vi "DataFinder Find Run Results.vi"(10 "RUNSELECT (Most Recent, First, ALL)":string, 11 "Run Results (empty)":T1[](array[typedef])) -> (3 "Filtered Run Results":T1[](array[typedef]))   [LabVIEW 2011]
uses:
  www/cgi-bin/_cgi-lib/TDM_INDEX Record.ctl
  www/cgi-bin/_cgi-lib/TDM_INDEX Record text SN sort.ctl
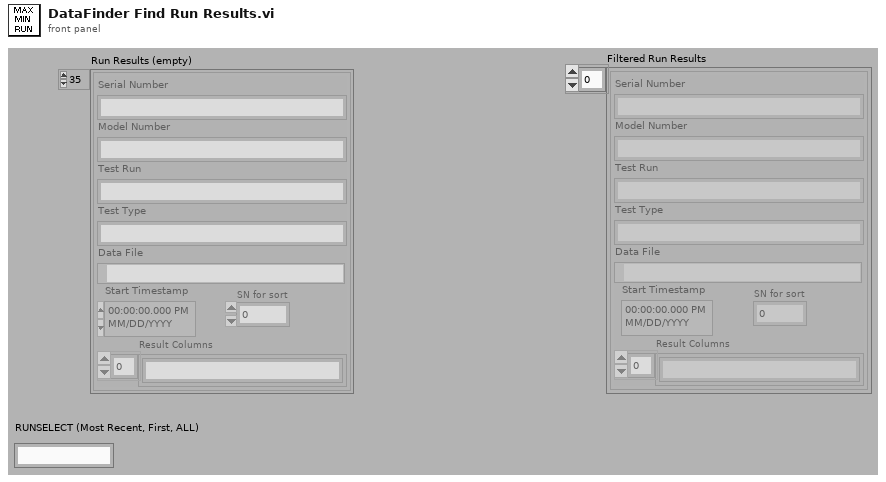
[diagram p1: front panel]
types:
  T1 = typedef "TDM_INDEX Record.ctl" = cluster{"Model Number":string, "SN for sort":i32, "Test Type":string, "Test Run":string, "Serial Number":string, "Start Timestamp":timestamp, "Data File":path, "Result Columns":string[]}
  T2 = typedef "TDM_INDEX Record text SN sort.ctl" = cluster{"Model Number":string, "Serial Number":string, "Test Type":string, "Test Run":string, "SN for sort":i32, "Start Timestamp":timestamp, "Data File":path, "Result Columns":string[]}
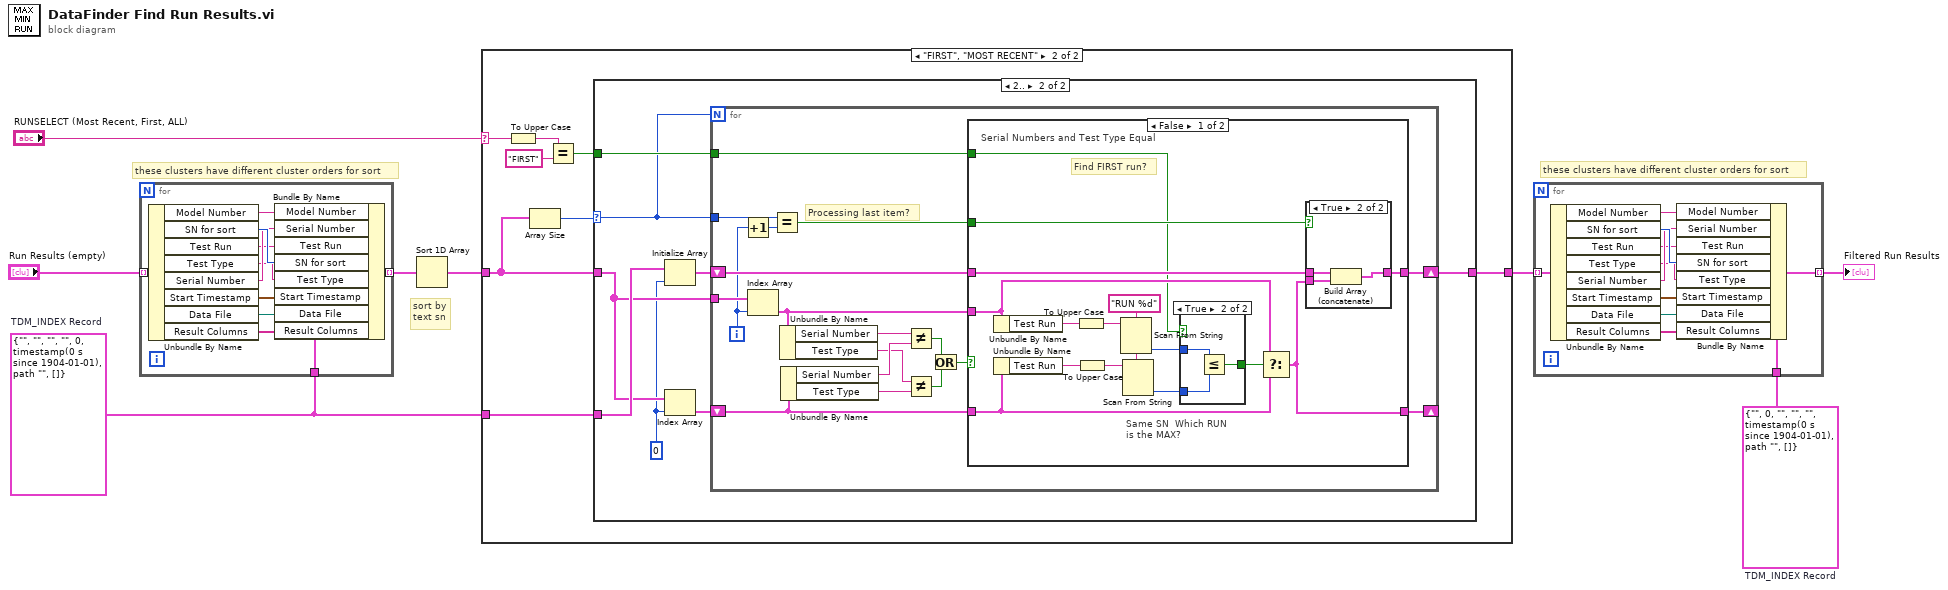
[diagram p0: block diagram]
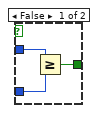
[diagram p4: hidden frame]
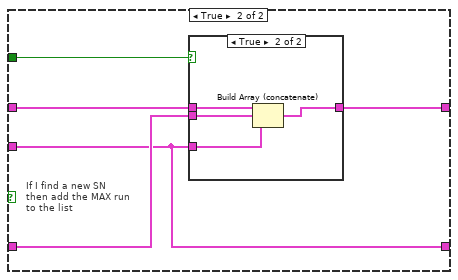
[diagram p6: hidden frame]
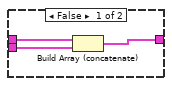
[diagram p7: hidden frame]
diagram:
  w3 = T1 {"Model Number"="", "SN for sort"=0, "Test Type"="", "Test Run"="", "Serial Number"="", "Start Timestamp"=timestamp(0 s since 1904-01-01), "Data File"=path "", "Result Columns"=[]}  # TDM_INDEX Record
  w6 = T2 {"Model Number"="", "Serial Number"="", "Test Type"="", "Test Run"="", "SN for sort"=0, "Start Timestamp"=timestamp(0 s since 1904-01-01), "Data File"=path "", "Result Columns"=[]}  # TDM_INDEX Record
  # "sort by\ntext sn"
  # "these clusters have different cluster orders for sort"
  # "these clusters have different cluster orders for sort"
  n1 = for {
    tunnel: "Run Results (empty)" -> [w19] mode=indexing
    tunnel: w6 -> [w18]
    tunnel: [w9] -> w5 mode=indexing
    n2 = Unbundle By Name(w19) -> ("Model Number"=w17:string, "SN for sort"=w16:i32, "Test Run"=w14:string, "Test Type"=w13:string, "Serial Number"=w15:string, "Start Timestamp"=w12:timestamp, "Data File"=w11:path, "Result Columns"=w10:string[])
    n3 = Bundle By Name(cluster=w18, "Model Number"=w17, "Serial Number"=w15, "Test Run"=w14, "SN for sort"=w16, "Test Type"=w13, "Start Timestamp"=w12, "Data File"=w11, "Result Columns"=w10) -> (w9:T2)
  }
  n4 = Sort 1D Array(array=w5) -> (sorted array=w4:T2[])
  n5 = case shown="\"FIRST\", \"MOST RECENT\"" "RUNSELECT (Most Recent, First, ALL)" {
    selector: "RUNSELECT (Most Recent, First, ALL)" -> [_ w24]
    tunnel: [w20 w28] -> w7
    tunnel: w4 -> [w20 w27]
    tunnel: w6 -> [_ w25]
    frame "ALL", Default {
    }
    frame "FIRST", "MOST RECENT" {
      n6 = To Upper Case(1:w24) -> (0:w21:string)
      n7 = Array Size(array=w27) -> (size(s)=w26:i32)
      n8 = Equal?(x=w21, y="FIRST") -> (x = y?=w22:bool)
      n9 = case shown="2.." w26 {
        selector: w26 -> [_ w31]
        tunnel: w25 -> [_ w37]
        tunnel: [w29 w35] -> w28
        tunnel: w27 -> [w29 w34]
        tunnel: w22 -> [_ w32]
        frame Default {
          # "If there are 0 or 1 elements no filtering is needed."
        }
        frame 2.. {
          w30 = 0
          n10 = Initialize Array(w37, w30) -> (w36:T2[])
          n11 = Index Array(array=w34, index=w30) -> (element=w33:T2)
          n12 = for {
            N: w31 -> [_]
            shift-right: [w54] -> w35
            shift-left: w36 -> [w55]
            tunnel: w34 -> [w51]
            shift-right: [w52] -> _
            shift-left: w33 -> [w48]
            tunnel: w31 -> [w39]
            tunnel: w32 -> [w40]
            i -> [w46]
            # "Processing last item?"
            n13 = Increment(x=w46) -> (x+1=w38:i32)
            n14 = Index Array(array=w51, index=w46) -> (element=w50:T2)
            n15 = Equal?(x=w39, y=w38) -> (x = y?=w49:bool)
            n16 = Unbundle By Name(w50) -> ("Serial Number"=w53:string, "Test Type"=w43:string)
            n17 = Unbundle By Name(w48) -> ("Serial Number"=w47:string, "Test Type"=w42:string)
            n18 = Not Equal?(x=w53, y=w47) -> (x != y?=w45:bool)
            n19 = Not Equal?(x=w43, y=w42) -> (x != y?=w41:bool)
            n20 = Or(x=w45, y=w41) -> (x .or. y?=w44:bool)
            n21 = case shown="False" w44 {
              tunnel: w55 -> [w64 w85]
              tunnel: [w65 w84] -> w54
              tunnel: w48 -> [w60 w83]
              tunnel: [w59 w81] -> w52
              tunnel: w50 -> [w61 w81]
              tunnel: w49 -> [w63 w82]
              tunnel: w40 -> [w56 _]
              frame False {
                w68 = "RUN %d" ("format string")
                # "Find FIRST run?"
                # "Serial Numbers and Test Type Equal"
                # "Same SN  Which RUN\nis the MAX?"
                n22 = Unbundle By Name(w61) -> ("Test Run"=w69:string)
                n23 = Unbundle By Name(w60) -> ("Test Run"=w70:string)
                n24 = To Upper Case(1:w69) -> (0:w58:string)
                n25 = To Upper Case(1:w70) -> (0:w57:string)
                n26 = Scan From String(format string=w68, input string=w58) -> (output 1=w67:i32)  [unwired: 2 in, 4 out]
                n27 = Scan From String(format string=w68, input string=w57) -> (output 1=w66:i32)  [unwired: 2 in, 4 out]
                n28 = case shown="True" w56 {
                  tunnel: w67 -> [w73 w76]
                  tunnel: w66 -> [w72 w75]
                  tunnel: [w71 w74] -> w62
                  frame False {
                    n29 = Greater Or Equal?(x=w73, y=w72) -> (x >= y?=w71:bool)
                  }
                  frame True {
                    n30 = Less Or Equal?(x=w76, y=w75) -> (x <= y?=w74:bool)
                  }
                }
                n31 = Select(t=w61, s=w62, f=w60) -> (s? t:f=w59:T2)
                n32 = case shown="True" w63 {
                  tunnel: [w77 w80] -> w65
                  tunnel: w64 -> [w77 w79]
                  tunnel: w59 -> [_ w78]
                  frame False {
                  }
                  frame True {
                    n33 = Build Array (concatenate)(w79, w78) -> (w80:T2[])
                  }
                }
              }
              frame True {
                # "If I find a new SN\nthen add the MAX run\nto the list"
                n34 = case shown="True" w82 {
                  tunnel: w85 -> [w88 w92]
                  tunnel: [w86 w91] -> w84
                  tunnel: w83 -> [w87 w90]
                  tunnel: w81 -> [_ w89]
                  frame False {
                    n35 = Build Array (concatenate)(w88, w87) -> (w86:T2[])
                  }
                  frame True {
                    n36 = Build Array (concatenate)(w92, w90, w89) -> (w91:T2[])
                  }
                }
              }
            }
          }
        }
      }
    }
  }
  n37 = for {
    tunnel: w7 -> [w103] mode=indexing
    tunnel: w3 -> [w102]
    tunnel: [w93] -> w2 mode=indexing
    n38 = Unbundle By Name(w103) -> ("Model Number"=w101:string, "SN for sort"=w100:i32, "Test Run"=w98:string, "Test Type"=w97:string, "Serial Number"=w99:string, "Start Timestamp"=w96:timestamp, "Data File"=w95:path, "Result Columns"=w94:string[])
    n39 = Bundle By Name(cluster=w102, "Model Number"=w101, "Serial Number"=w99, "Test Run"=w98, "SN for sort"=w100, "Test Type"=w97, "Start Timestamp"=w96, "Data File"=w95, "Result Columns"=w94) -> (w93:T1)
  }
  "Filtered Run Results" <- w2
